vi "gh-cli Auth Login.vi"(8 "error in (no error)":errorcluster, 11 "Git in":refnum<class "Git.lvclass">) -> (0 "error out":errorcluster, 3 "Git out":refnum<class "Git.lvclass">)   [LabVIEW 2019, in "Git.lvclass"]
doc: "gh auth login: Authenticate with a GitHub host. The default authentication mode is a web-based browser flow. After completion, an authentication token will be stored internally.\n\n<b>Important</b>: This VI will not wait until completion in order to allow the user to interact with the command prompt.\n\nhttps://cli.github.com/manual"
uses:
  Git.lvclass
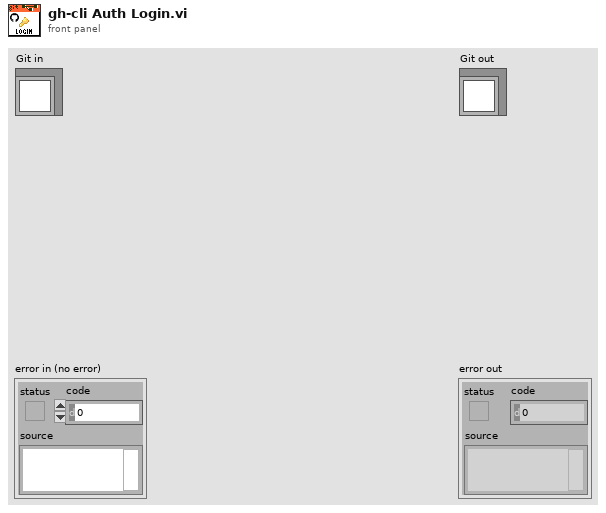
[diagram p1: front panel]
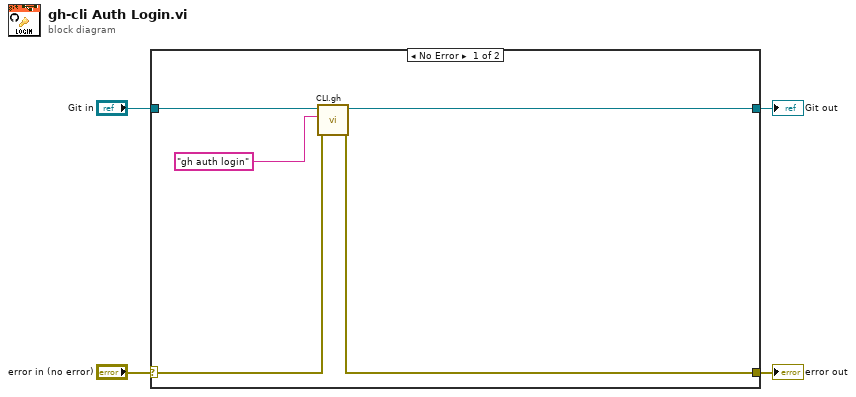
[diagram p0: block diagram]
diagram:
  n1 = case shown="No Error" "error in (no error)" {
    selector: "error in (no error)" -> [w7 w11]
    tunnel: [w6 w11] -> w3
    tunnel: [w8 w10] -> w1
    tunnel: "Git in" -> [w9 w10]
    frame No Error {
      n2 = call "CLI.gh.vi"("error in (no error)"=w7, "Command"="gh auth login", "Git in"=w9) -> ("error out"=w6:errorcluster, "Git out"=w8:refnum<class "Git.lvclass">)  [unwired: 4 in, 3 out]
    }
    frame Error {
    }
  }
  "error out" <- w3
  "Git out" <- w1
